vi "List.vi"() -> ()   [LabVIEW 2021]
uses:
  <userlib>/SciSDK/SciSDK_Labview.lvlib
panel:
  out "Counter":i8
  out "CH0":i8
  out "CH1":i8
  out "List Buffer Out":T1
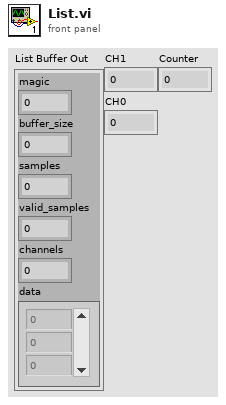
[diagram p1: front panel]
types:
  T1 = cluster{"magic":u32, "buffer_size":u32, "samples":u32, "valid_samples":u32, "channels":u32, "data":i8[]}
  T2 = cluster{"Name":string, "Board Model":string, "Handle":u64}
  T3 = cluster{"Board Name":string, "Board Model":string, "Handle":u64}
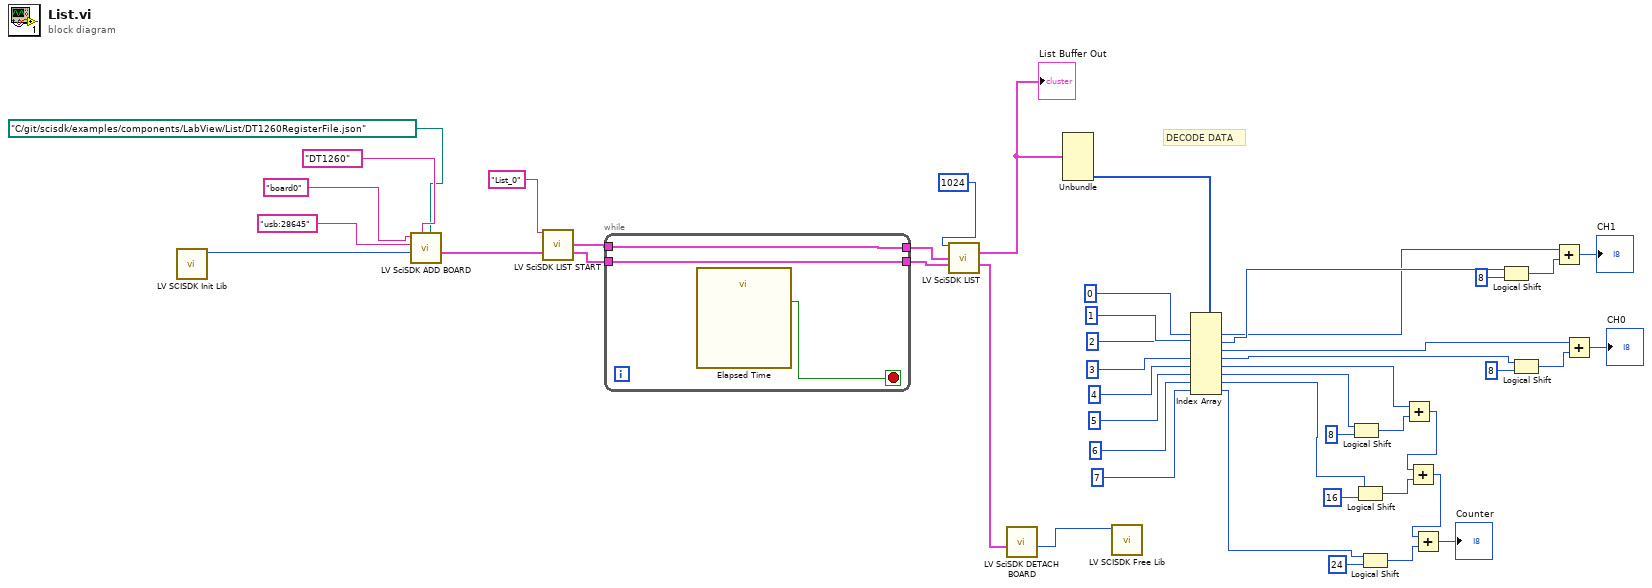
[diagram p0: block diagram]
diagram:
  # "DECODE DATA"
  n1 = call <userlib>:"LV SCISDK Init Lib.vi"() -> ("function return"=w47:u64)  [unwired: 11 in]
  n2 = call <userlib>:"LV SciSDK ADD BOARD.vi"("JsonFile"=path "C:/git/scisdk/examples/components/LabView/List/DT1260RegisterFile.json", "Board Model"="DT1260", "SciSDK Handle"=w47, "DevicePath"="usb:28645", "Name"="board0") -> ("Board Handle Out"=w42:T2)  [unwired: 4 in, 2 out]
  n3 = call <userlib>:"LV SciSDK LIST START.vi"("List name"="List_0", "Handle In"=w42) -> ("CP Handle Out"=w39:cluster{"CP Path":string, "CP Name":string}, "Handle Out"=w40:T3)  [unwired: 15 in, 1 out]
  n4 = while {
    tunnel: w39 -> [w49]
    tunnel: w40 -> [w48]
    tunnel: [w49] -> w37
    tunnel: [w48] -> w36
    stop <- w50 stop-if-true
    n5 = call "Elapsed Time"() -> ("Time has Elapsed"=w50:bool)  [unwired: 12 in, 7 out]
  }
  n6 = call <userlib>:"LV SciSDK LIST.vi"("Buffer Size"=u32 1024, "List Handle In"=w37, "Board Handle In"=w36) -> ("List Buffer Out"=w35:T1, "Board Handle Out"=w1:T3)  [unwired: 8 in, 3 out]
  "List Buffer Out" <- w35
  n7 = call <userlib>:"LV SciSDK DETACH BOARD.vi"("Board Handle In"=w1) -> ("SciSDK Handle"=w2:u64)  [unwired: 9 in, 1 out]
  n8 = Unbundle(w35) -> ("data"=w34:i8[])  [unwired: 5 out]
  n9 = call <userlib>:"LV SCISDK Free Lib.vi"("handle"=w2) -> ()  [unwired: 9 in, 2 out]
  n10 = Index Array(array=w34, index #1=0 ("index"), index #2=1 ("index"), index #3=2 ("index"), index #4=3 ("index"), index #5=4 ("index"), index #6=5 ("index"), index #7=6 ("index"), index #8=7 ("index")) -> (element #1=w23:i8, element #2=w25:i8, element #3=w17:i8, element #4=w16:i8, element #5=w9:i8, element #6=w7:i8, element #7=w6:i8, element #8=w5:i8)
  n11 = Logical Shift(y=w7, x=i8 8) -> (x << y=w14:i8)
  n12 = Logical Shift(y=w6, x=i8 16) -> (x << y=w12:i8)
  n13 = Logical Shift(y=w5, x=i8 24) -> (x << y=w10:i8)
  n14 = Add(x=w9, y=w14) -> (x+y=w8:i8)
  n15 = Add(x=w8, y=w12) -> (x+y=w4:i8)
  n16 = Add(x=w4, y=w10) -> (x+y=→"Counter":i8)
  n17 = Logical Shift(y=w25, x=i8 8) -> (x << y=w22:i8)
  n18 = Logical Shift(y=w16, x=i8 8) -> (x << y=w19:i8)
  n19 = Add(x=w23, y=w22) -> (x+y=→"CH1":i8)
  n20 = Add(x=w17, y=w19) -> (x+y=→"CH0":i8)
